vi "Get Children.vi"(8 "error in (no error)":errorcluster, 11 "Element in":refnum<class "Element.lvclass">) -> (0 "error out":errorcluster, 2 "Children":refnum<class "Data Item.lvclass">[](array[class]), 3 "Element out":refnum<class "Element.lvclass">)   [LabVIEW 2023, in "VILab.lvlib" / "Element.lvclass"]
uses:
  Element.lvclass
  Data Item/Data Item.lvclass
  Element.lvclass/Element.ctl
  Attribute/Attribute.lvclass
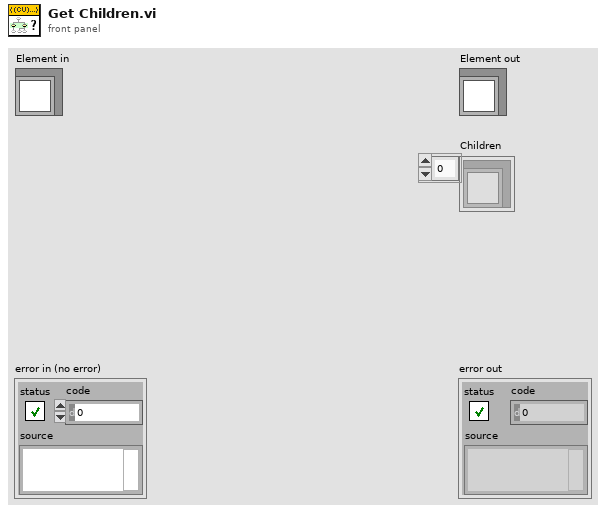
[diagram p1: front panel]
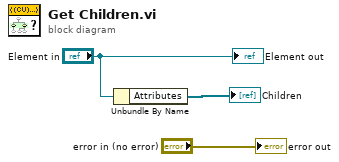
[diagram p0: block diagram]
diagram:
  n1 = Unbundle By Name("Element in") -> ("Attributes"=→"Children":refnum<class "Attribute.lvclass">[])
  "error out" <- "error in (no error)"
  "Element out" <- "Element in"
